vi "Spatial Dual Decode Packet 40 (SubVI).vi"(8 "SGL Precision":i16=6, 10 "Packet 40 Bytes In":u8[](array[numeric])) -> (0 "Channel Data Type":string[](array[string])=["Float", "Float", "Float"], 1 "Channel Units":string[](array[string])=["m/s/s", "m/s/s", "m/s/s"], 2 "Data":string[](array[string]), 3 "Channel Names":string[](array[string])=["Acc X", "Acc Y", "Acc Z"], 4 "Packet 40 Decoded Data Cluster":cluster{"QS":sgl, "QX":sgl, "QY":sgl, "QZ":sgl})   [LabVIEW 2019, in "SpatialDual_Parsers.lvlib"]
uses:
  SpatialDual_Parsers.lvlib
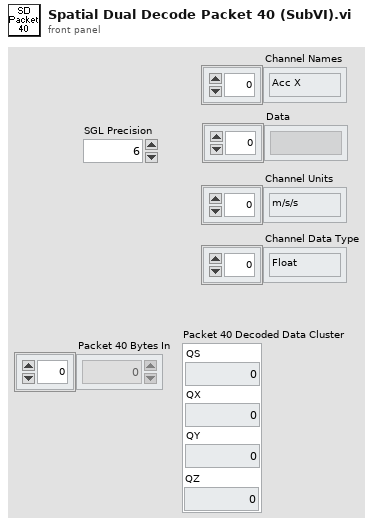
[diagram p1: front panel]
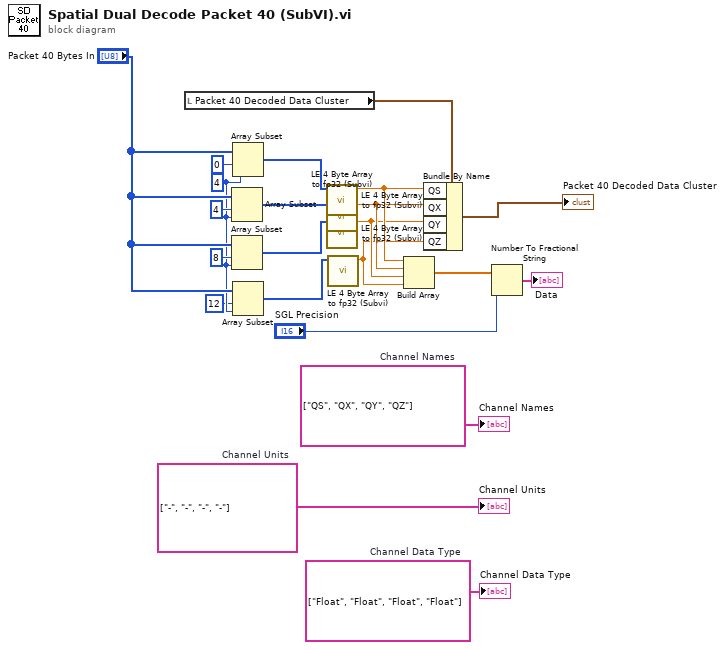
[diagram p0: block diagram]
diagram:
  w6 = string[] ["Float", "Float", "Float", "Float"]  # Channel Data Type
  w7 = string[] ["-", "-", "-", "-"]  # Channel Units
  w8 = string[] ["QS", "QX", "QY", "QZ"]  # Channel Names
  w4 = 4 ("length")
  n1 = local read "Packet 40 Decoded Data Cluster"() -> (w22:cluster{"QS":sgl, "QX":sgl, "QY":sgl, "QZ":sgl})
  n2 = Array Subset(array="Packet 40 Bytes In", index=4, length=w4) -> (w16:u8[])
  n3 = Array Subset(array="Packet 40 Bytes In", index=8, length=w4) -> (w17:u8[])
  n4 = Array Subset(array="Packet 40 Bytes In", index=0, length=w4) -> (w15:u8[])
  n5 = Array Subset(array="Packet 40 Bytes In", index=12, length=w4) -> (w2:u8[])
  n6 = call "LE 4 Byte Array to fp32 (Subvi).vi"("4 Bytes in"=w15) -> ("fp32 Out"=w14:sgl)  [unwired: 8 in]
  n7 = call "LE 4 Byte Array to fp32 (Subvi).vi"("4 Bytes in"=w16) -> ("fp32 Out"=w13:sgl)  [unwired: 8 in]
  n8 = call "LE 4 Byte Array to fp32 (Subvi).vi"("4 Bytes in"=w17) -> ("fp32 Out"=w12:sgl)  [unwired: 8 in]
  n9 = call "LE 4 Byte Array to fp32 (Subvi).vi"("4 Bytes in"=w2) -> ("fp32 Out"=w1:sgl)  [unwired: 8 in]
  n10 = Build Array(w14, w13, w12, w1) -> (w11:sgl[])
  n11 = Bundle By Name(cluster=w22, "QS"=w14, "QX"=w13, "QY"=w12, "QZ"=w1) -> (→"Packet 40 Decoded Data Cluster":cluster{"QS":sgl, "QX":sgl, "QY":sgl, "QZ":sgl})
  n12 = Number To Fractional String(number=w11, precision (6)="SGL Precision") -> (F-format string=→"Data":string[])  [unwired: 2 in]
  "Channel Names" <- w8
  "Channel Units" <- w7
  "Channel Data Type" <- w6
